vi "Is Project Control.vi"(8 "error in (no error)":errorcluster, 10 "Project":refnum<class "Project.lvclass">, 11 "Control Value":variant) -> (0 "error out":errorcluster, 3 "Is Project Control":bool)   [LabVIEW 2015, in "CallVIStep.lvclass"]
uses:
  CallVIStep.lvclass
  Project.lvclass
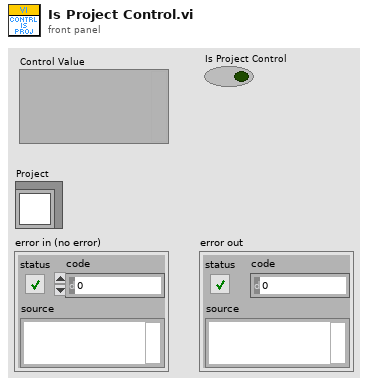
[diagram p1: front panel]
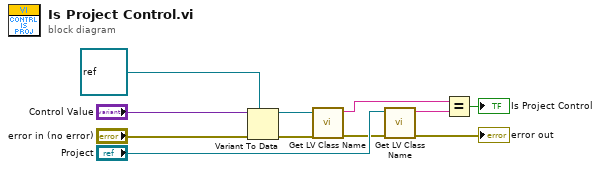
[diagram p0: block diagram]
diagram:
  n1 = Variant To Data(error in="error in (no error)", type=refnum<class> refnum ("LabVIEW Object"), Variant="Control Value") -> (data=w4:refnum<class>, error out=w5:errorcluster)
  n2 = call <vilib>:"Get LV Class Name.vi"("error in (no error)"=w5, "object"=w4) -> ("error out"=w6:errorcluster, "class name"=w7:string)  [unwired: 8 in]
  n3 = call <vilib>:"Get LV Class Name.vi"("error in (no error)"=w6, "object"="Project") -> ("error out"=→"error out":errorcluster, "class name"=w8:string)  [unwired: 8 in]
  n4 = Equal?(x=w7, y=w8) -> (x = y?=→"Is Project Control":bool)
